vi "sub random leds.vi"() -> (0 "concatenated string":string)   [LabVIEW 2016]
panel:
  out "Array 2":u16[][](array[ring])
  out "string":string
  out "Array":dbl[](array[numeric])
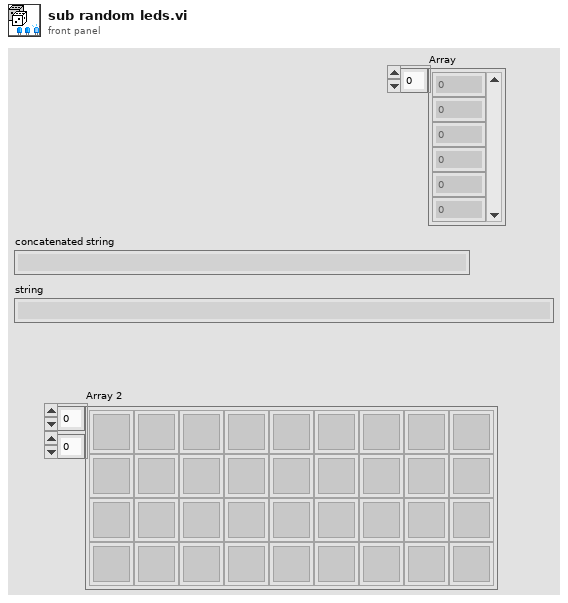
[diagram p1: front panel]
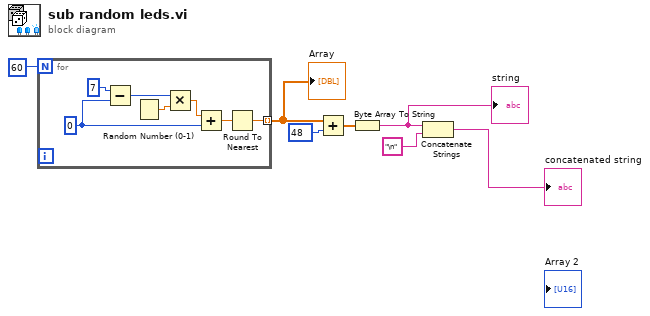
[diagram p0: block diagram]
diagram:
  n1 = for {
    N: 60 -> [_]
    tunnel: [w9] -> w6 mode=indexing
    w11 = u8 0 ("MIN")
    n2 = Subtract(x=u8 7 ("MAX"), y=w11) -> (x-y=w13:u8)
    n3 = Random Number (0-1)() -> (number: 0 to 1=w8:dbl)
    n4 = Multiply(x=w13, y=w8) -> (x*y=w12:dbl)
    n5 = Add(x=w12, y=w11) -> (x+y=w10:dbl)
    n6 = Round To Nearest(number=w10) -> (nearest integer value=w9:dbl)
  }
  "Array" <- w6
  n7 = Add(x=w6, y=u8 48) -> (x+y=w4:dbl[])
  n8 = Byte Array To String(unsigned byte array=w4) -> (string=w3:string)
  "string" <- w3
  n9 = Concatenate Strings(w3, "\n" ("string")) -> (→"concatenated string":string)
